vi "Check endstop str.vi"(8 "error in (no error)":errorcluster, 10 "Ens-stop state in":bool[](array[boolean]), 11 "Data in":string) -> (0 "error out":errorcluster, 2 "Ens-stop state out":bool[](array[boolean]))   [LabVIEW 2020, in "Control de MaP.lvlib"]
uses:
  Control de MaP.lvlib
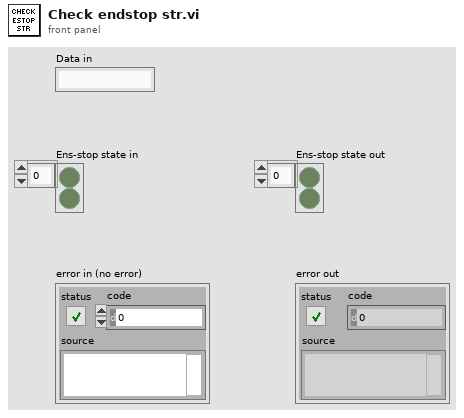
[diagram p1: front panel]
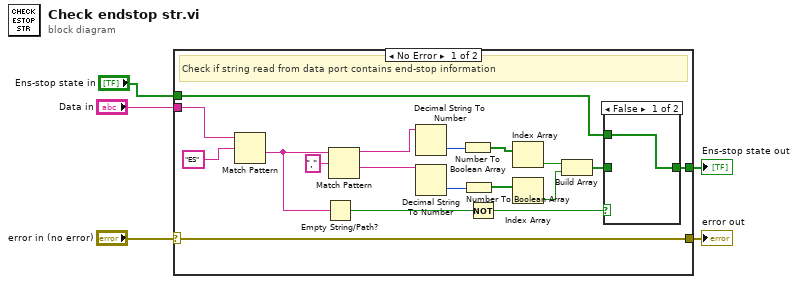
[diagram p0: block diagram]
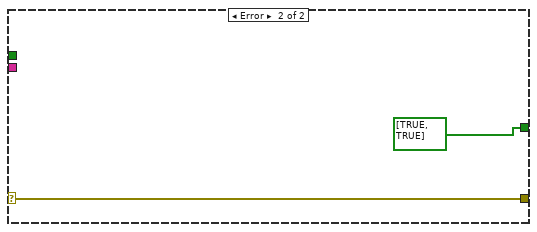
[diagram p3: hidden frame]
diagram:
  n1 = case shown="No Error" "error in (no error)" {
    selector: "error in (no error)" -> [w11 w27]
    tunnel: "Data in" -> [w21 _]
    tunnel: [w8 bool[] [TRUE, TRUE]] -> w4
    tunnel: [w11 w27] -> w2
    tunnel: "Ens-stop state in" -> [w7 _]
    frame No Error {
      # "Check if string read from data port contains end-stop information"
      n2 = Match Pattern(string=w21, regular expression="ES") -> (after substring=w20:string)  [unwired: 1 in, 3 out]
      n3 = Empty String/Path?(string/path=w20) -> (empty?=w10:bool)
      n4 = Match Pattern(string=w20, regular expression=",") -> (before substring=w19:string, after substring=w18:string)  [unwired: 1 in, 2 out]
      n5 = Decimal String To Number(string=w19) -> (number=w17:i32)  [unwired: 2 in, 1 out]
      n6 = Decimal String To Number(string=w18) -> (number=w16:i32)  [unwired: 2 in, 1 out]
      n7 = Number To Boolean Array(number=w17) -> (Boolean array=w15:bool[])
      n8 = Number To Boolean Array(number=w16) -> (Boolean array=w14:bool[])
      n9 = Not(x=w10) -> (.not. x?=w6:bool)
      n10 = Index Array(array=w15) -> (element=w13:bool)  [unwired: 1 in]
      n11 = Index Array(array=w14) -> (element=w12:bool)  [unwired: 1 in]
      n12 = Build Array(w13, w12) -> (w9:bool[])
      n13 = case shown="False" w6 {
        tunnel: w9 -> [_ w25]
        tunnel: [w24 w25] -> w8
        tunnel: w7 -> [w24 _]
        frame False {
        }
        frame True {
        }
      }
    }
    frame Error {
    }
  }
  "error out" <- w2
  "Ens-stop state out" <- w4
